vi "AIT 664 - Match Parameters Input VL.vi"(0 "664 End System Parameter File":T5, 5 "664 End System Configuration File":T5, 11 "error in":errorcluster) -> (4 "Input VLs out":T1[](array[typedef]), 15 "error out":errorcluster)   [LabVIEW 2013, in "AIT 664 Custom Device.lvlib"]
doc: "Match the Input VLs from xml file and parameter file."
uses:
  AIT 664 Custom Device.lvlib
  Controls/664 - XML End System Description.ctl
  Controls/664 - XML Output VL.ctl
  Controls/664 - XML Tx Message Port.ctl
  Controls/664 - Sampling Type.ctl
  Controls/664 -Param.ctl
  Controls/664 - XML Input VL.ctl
  Controls/664 - XML Rx Message Port.ctl
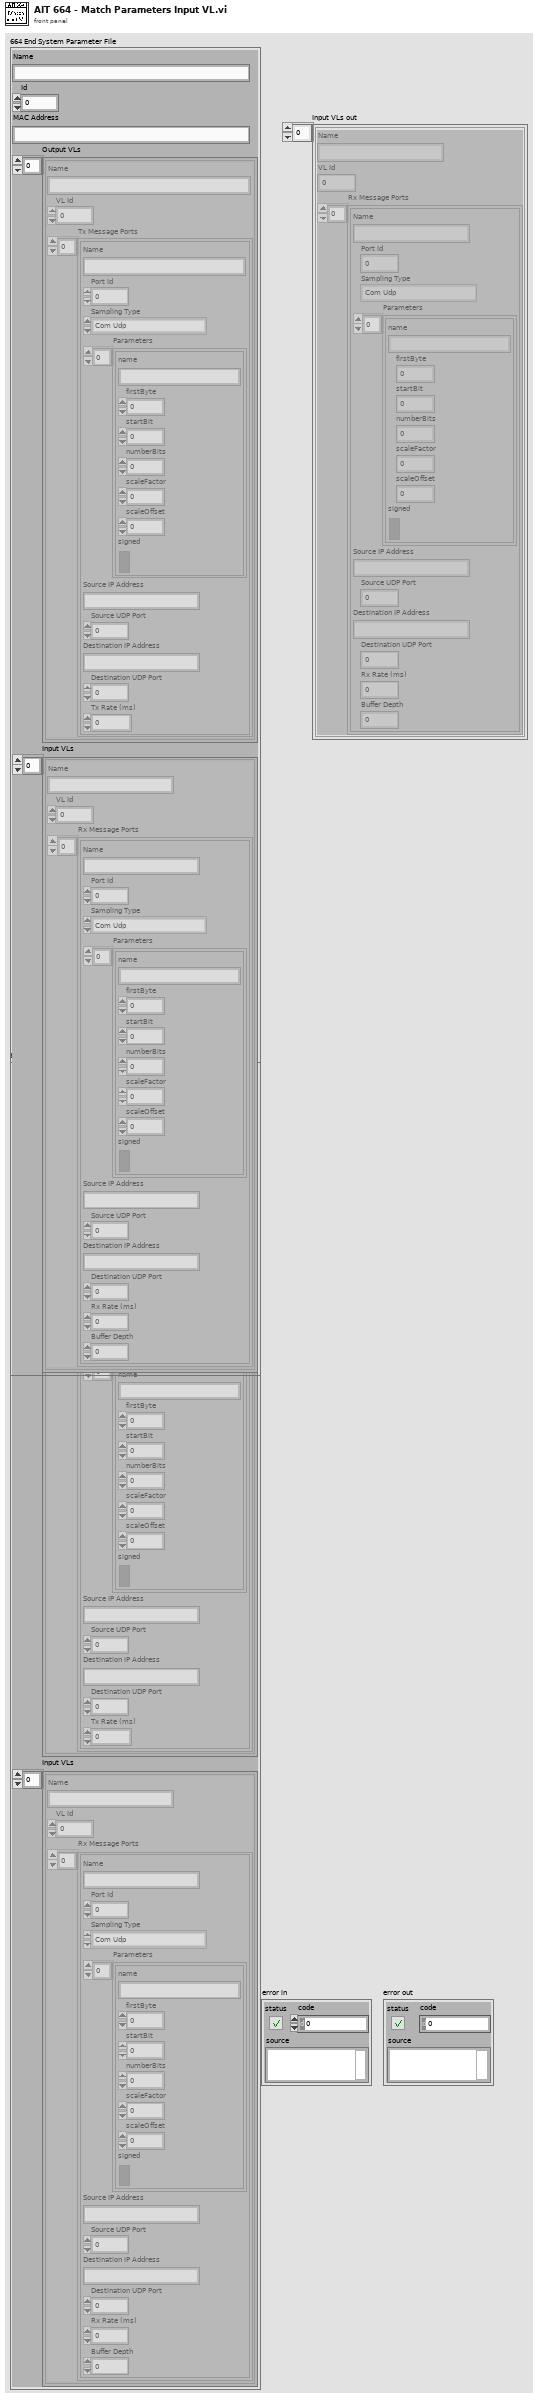
[diagram p1: front panel]
types:
  T1 = typedef "AIT 664 Custom Device.lvlib/664 - XML Input VL.ctl" = cluster{"Name":string, "VL Id":u32, "Rx Message Ports":T2[]}
  T2 = typedef "AIT 664 Custom Device.lvlib/664 - XML Rx Message Port.ctl" = cluster{"Name":string, "Port Id":u32, "Sampling Type":T3, "Parameters":T4[], "Source IP Address":string, "Source UDP Port":u32, "Destination IP Address":string, "Destination UDP Port":u32, "Rx Rate (ms)":u32, "Buffer Depth":u32}
  T3 = typedef "AIT 664 Custom Device.lvlib/664 - Sampling Type.ctl" = enum16{"Com Udp", "Com Udp Queuing", "Sap Udp", "Sap Ip", "Sap Mac", "Unknown"}
  T4 = typedef "AIT 664 Custom Device.lvlib/664 -Param.ctl" = cluster{"name":string, "firstByte":i32, "startBit":i32, "numberBits":i32, "scaleFactor":dbl, "scaleOffset":dbl, "signed":bool}
  T5 = typedef "AIT 664 Custom Device.lvlib/664 - XML End System Description.ctl" = cluster{"Name":string, "Id":u32, "MAC Address":string, "Output VLs":T6[], "Input VLs":T1[]}
  T6 = typedef "AIT 664 Custom Device.lvlib/664 - XML Output VL.ctl" = cluster{"Name":string, "VL Id":u32, "Tx Message Ports":T7[]}
  T7 = typedef "AIT 664 Custom Device.lvlib/664 - XML Tx Message Port.ctl" = cluster{"Name":string, "Port Id":u32, "Sampling Type":T3, "Parameters":T4[], "Source IP Address":string, "Source UDP Port":u32, "Destination IP Address":string, "Destination UDP Port":u32, "Tx Rate (ms)":u32}
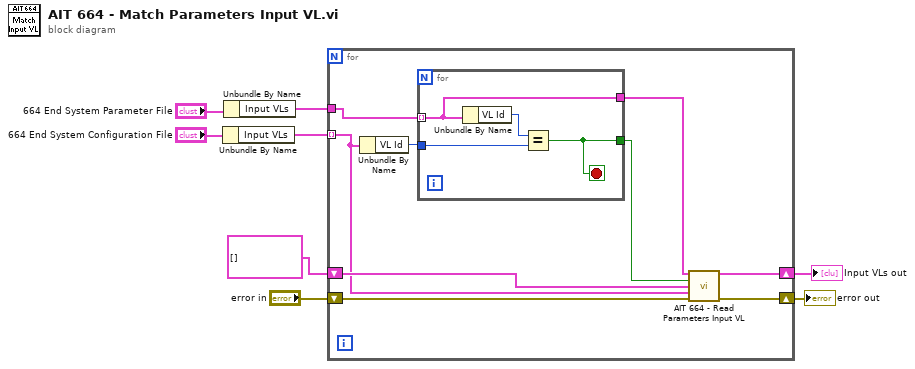
[diagram p0: block diagram]
diagram:
  n1 = Unbundle By Name("664 End System Configuration File") -> ("Input VLs"=w5:T1[])
  n2 = Unbundle By Name("664 End System Parameter File") -> ("Input VLs"=w3:T1[])
  n3 = for {
    tunnel: w5 -> [w12] mode=indexing
    tunnel: w3 -> [w17]
    shift-right: [w13] -> w6
    shift-left: T1[] [] -> [w14]
    shift-right: [w10] -> w2
    shift-left: "error in" -> [w9]
    n4 = Unbundle By Name(w12) -> ("VL Id"=w16:u32)
    n5 = for {
      tunnel: w17 -> [w18] mode=indexing
      tunnel: w16 -> [w20]
      tunnel: [w19] -> w15
      tunnel: [w18] -> w11
      stop <- w19 stop-if-true
      n6 = Unbundle By Name(w18) -> ("VL Id"=w21:u32)
      n7 = Equal?(x=w21, y=w20) -> (x = y?=w19:bool)
    }
    n8 = call "AIT 664 - Read Parameters Input VL.vi"("Input VL Parameter File"=w11, "Found VL?"=w15, "Input VLs"=w14, "Input VL Configuration File"=w12, "error in (no error)"=w9) -> ("Input VLs out"=w13:T1[], "error out"=w10:errorcluster)  [unwired: 9 in]
  }
  "Input VLs out" <- w6
  "error out" <- w2
